vi "ReadFromDB_labelconfig.vi"(0 "DB1":T1, 5 "操作模式":T2(ring)=enum."查询数据", 7 "查询项目":string="LuxsharePN,CustomerPN,Customer,SampleDes,AWG,Length,EEPROMWrite,LabelPrint,Remarks", 11 "标识列":string, 12 "限定条件":string="where LuxsharePN='L12345678'", 13 "Page":string, 15 "Desc":string) -> (14 "数据输出2":dbl[][](array[numeric]), 16 "错误类型":string, 17 "StringArray2":string[][](array[string])=[["L12345678\t\tIBM\t40G Ethernet QSFP+ Passive DAC Cable\t28\t3000\t0\t0\trefer to IBM Spec"]], 18 "列内对数":i32=1, 19 "返回记录数目":i32=1, 20 "ConvertToArray":string[][](array[string])=[["L12345678", "", "IBM", "40G Ethernet QSFP+ Passive DAC Cable", "28", "3000", "0", "0", "refer to IBM Spec"]], 21 "status":bool, 23 "ResultString":string="L12345678\t\tIBM\t40G Ethernet QSFP+ Passive DAC Cable\t28\t3000\t0\t0\trefer to IBM Spec\r", 24 "ConvertToClusterArray":cluster{"项":string, "值":string}[](array[cluster])=[{"项"="", "值"=""}, {"项"="L12345678", "值"="L12345678"}], 25 "DataPair":dbl[](array[numeric]), 27 "数据输出":dbl[][](array[numeric]))   [LabVIEW 2011]
uses:
  <vilib>/Utility/file.llb/Read From Spreadsheet File (string).vi
  <vilib>/Utility/file.llb/Write To Spreadsheet File (string).vi
panel:
  out "result string":string="select LuxsharePN,CustomerPN,Customer,SampleDes,AWG,Length,EEPROMWrite,LabelPrint,Remarks from project where LuxsharePN='L12345678'"
  out "替换数量":i32=9
  in  "二级分隔符":string
  in  "一级分隔符":string
  in  "表名":string="vproject"
  out "Result":bool=TRUE
  in  "InitArray1":string[][](array[string])
  in  "MoveToTail":i32=1
  in  "InitArray2":string[](array[string])
  out "错误输出":errorcluster
  in  "初始化簇数组":cluster{"项":string, "值":string}[](array[cluster])
  in  "簇元素":cluster{"项":string, "值":string}
  in  "input-db":string="HTPSDB"
  in  "input-psw":string="htps'songyy"
  in  "input-user":string="htpsuser"
  in  "input-IP":string="dg-sql-01.luxshare.com.cn"
  in  "ADODB._Recordset":refnum<k7>
  in  "ADODB._Connection":refnum<k7>
  # "列名 & 表名 查询结果"
  # "输       出"
  # "输       入"
  # "基本信息\n（）"
  # "状态灯，False表示操作成功，True表示操作失败"
  # "簇数组"
  # "限定条件，设定某个条件，输出满足该条件的数据"
  # "对数"
  # "错误类型"
  # "查询记录时才需要填写，page用于设置查询一次请求的记录数，Desc用于截断Desc条记录之前的记录"
  # "改变操作时需要修改的信息"
  # "操作模式：查询表名\n                  查询列名\n                  查询记录\n                  查询总记录\n                  查询数据"
  # "字符串"
  # "数组"
  # "查询表名时不需要输入\n\n查询列名和查询数据时要指定哪一张表"
  # "字符串数组"
  # "在查询表名和列名时不需要输入信息\n\n在查询数据时，如果要输入所有列，填入“*”，如果要查询指定的某一个列，输入该列的名称"
  # "ProjectName"
  # "EEPROMContent"
  # "LimitSpec"
  # "LabelContent"
  # "SwitchMatrix"
  # "error:\n-2147217843 登陆失败： 。\n-2147467259 要访问的数据库不存在\n-2146825267 没有数据    。\n-2146824584 对象关闭时，不允许操作\n-2147217865 表名不存在 。\n-2147467259 服务器连接失败 。"
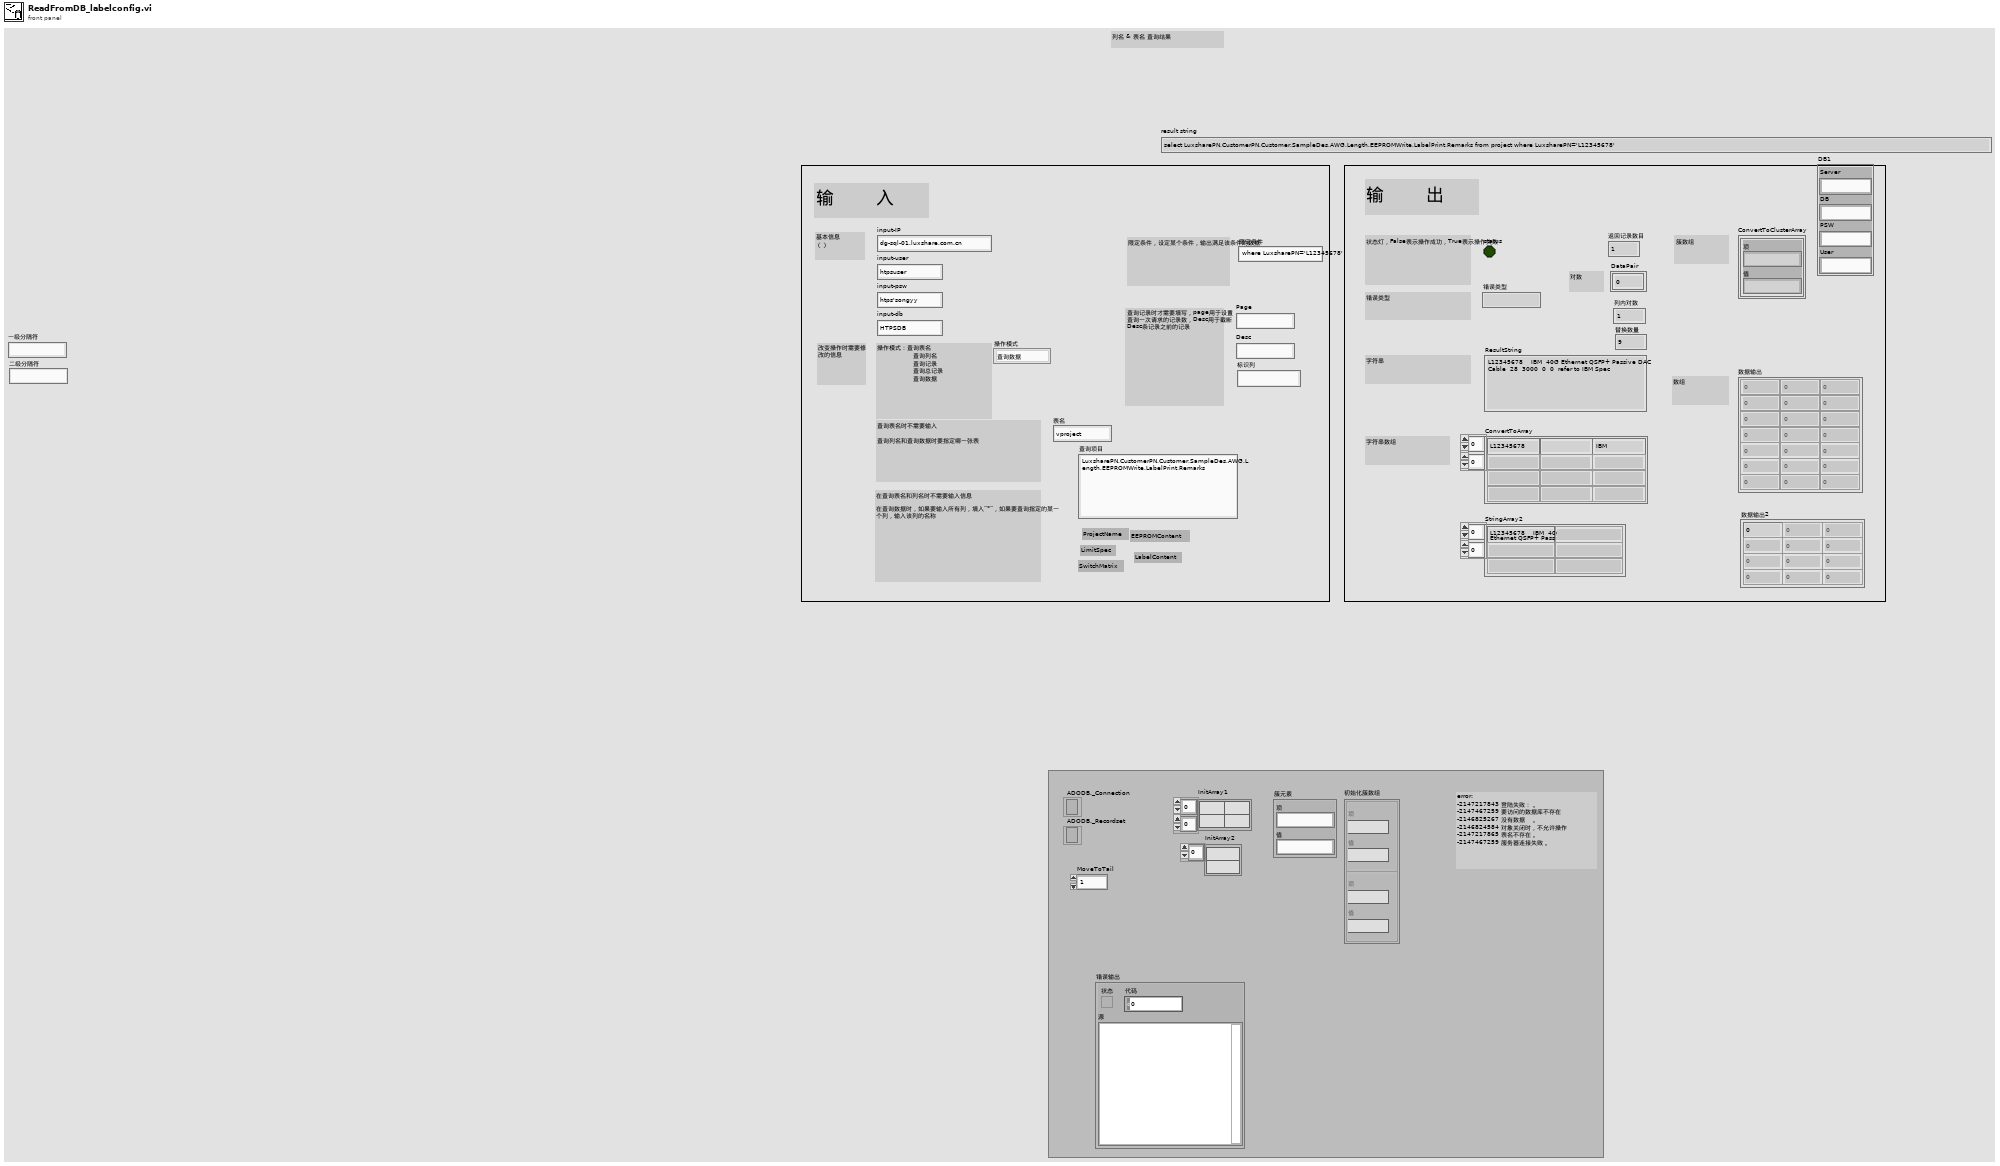
[diagram p1: front panel]
types:
  T1 = cluster{"Server":string, "DB":string, "PSW":string, "User":string}
  T2 = enum16{"查询表名", "查询列名", "查询记录", "查询总记录", "查询数据", "转换数据"}
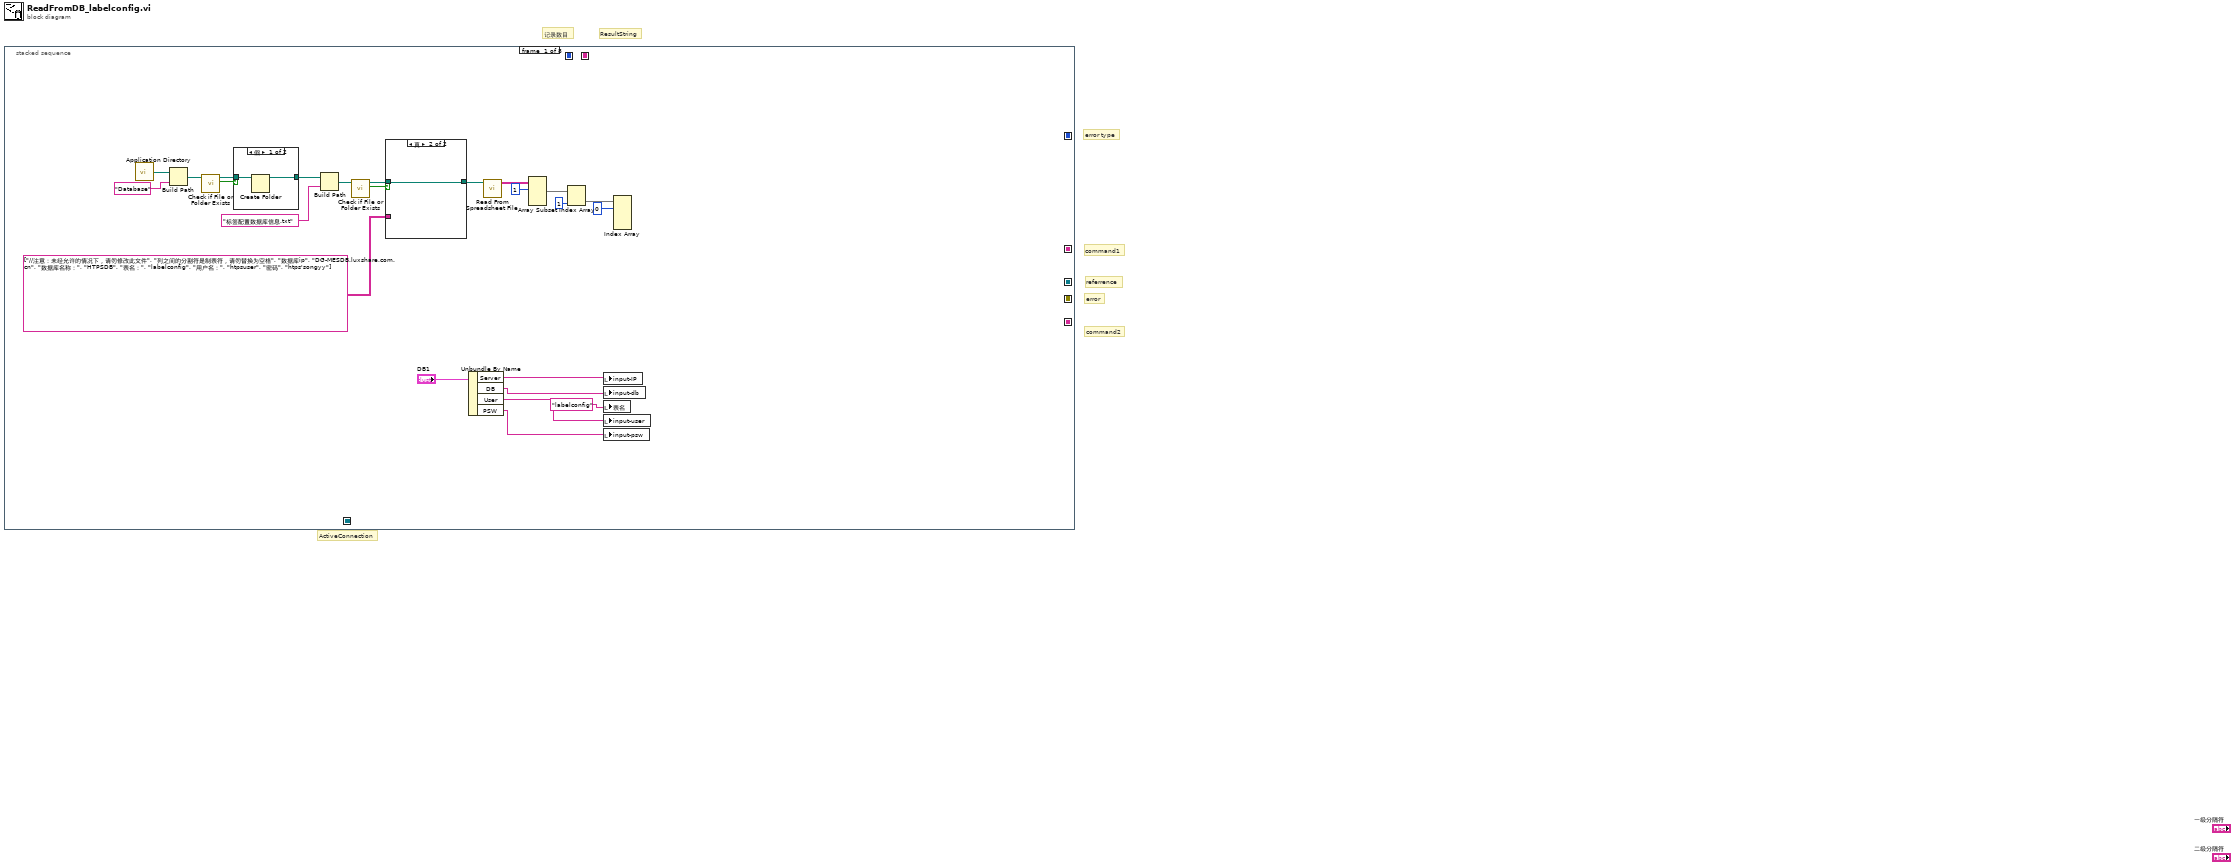
[diagram p0: block diagram]
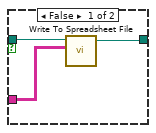
[diagram p2: hidden frame]
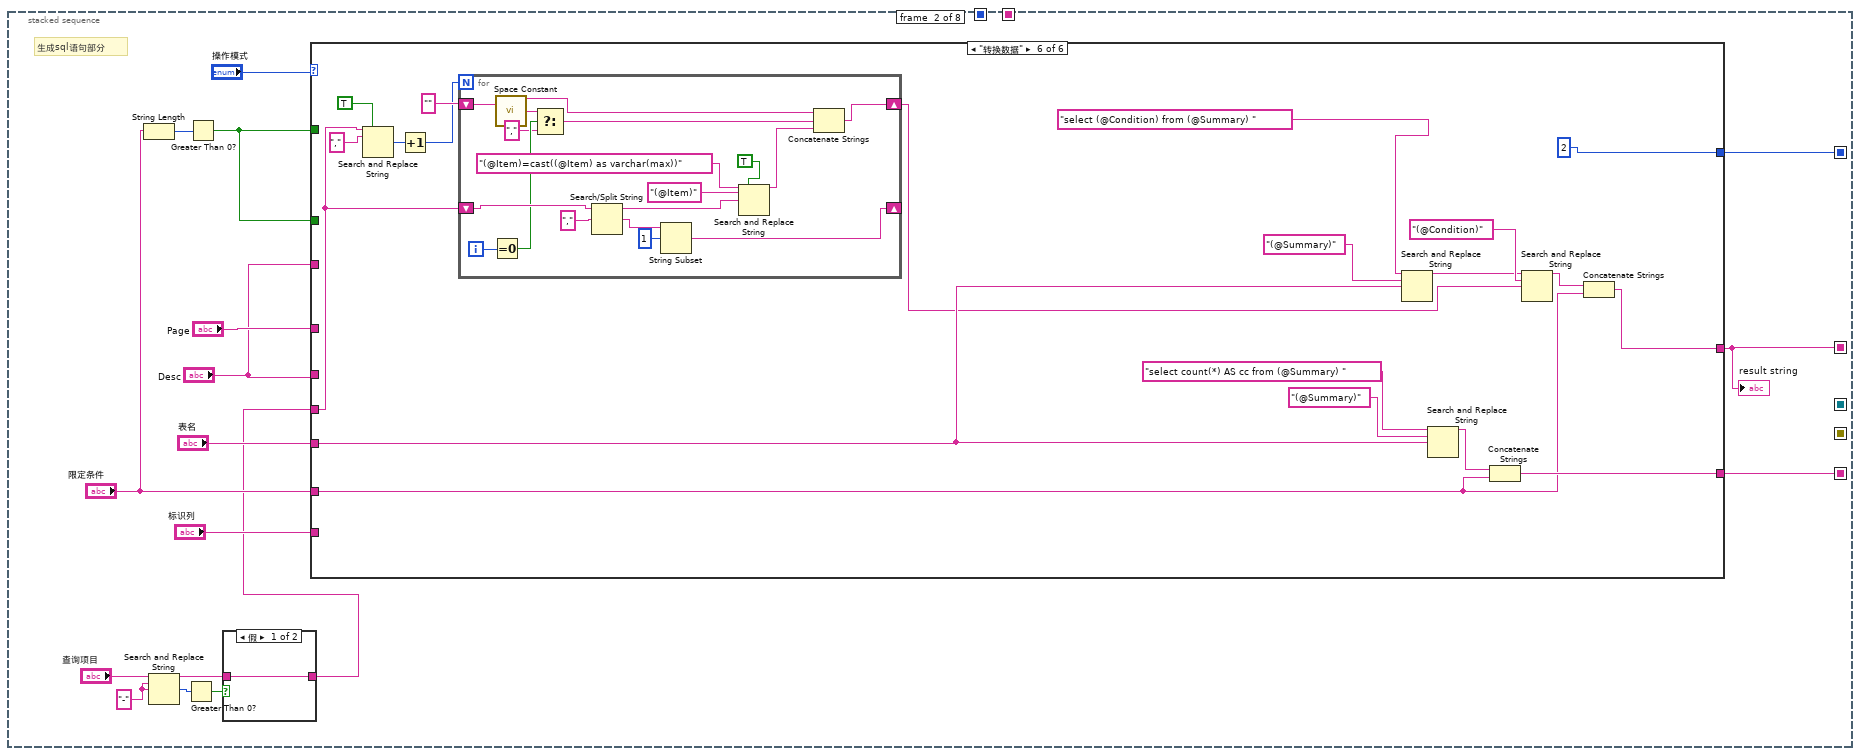
[diagram p4: hidden frame]
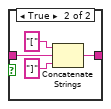
[diagram p5: hidden frame]
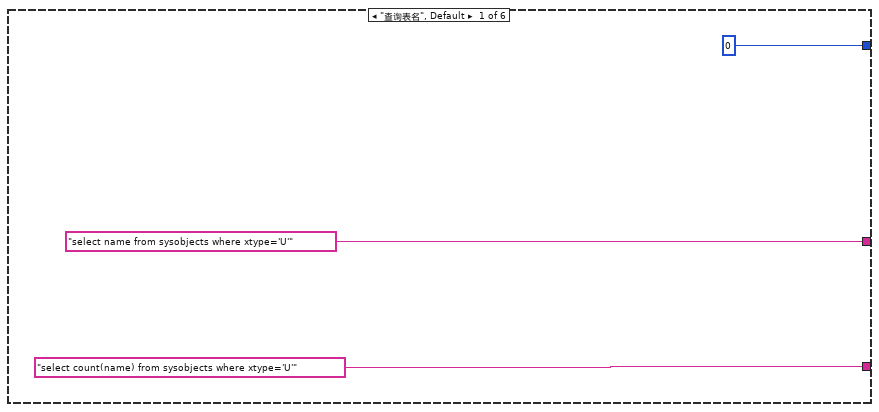
[diagram p6: hidden frame]
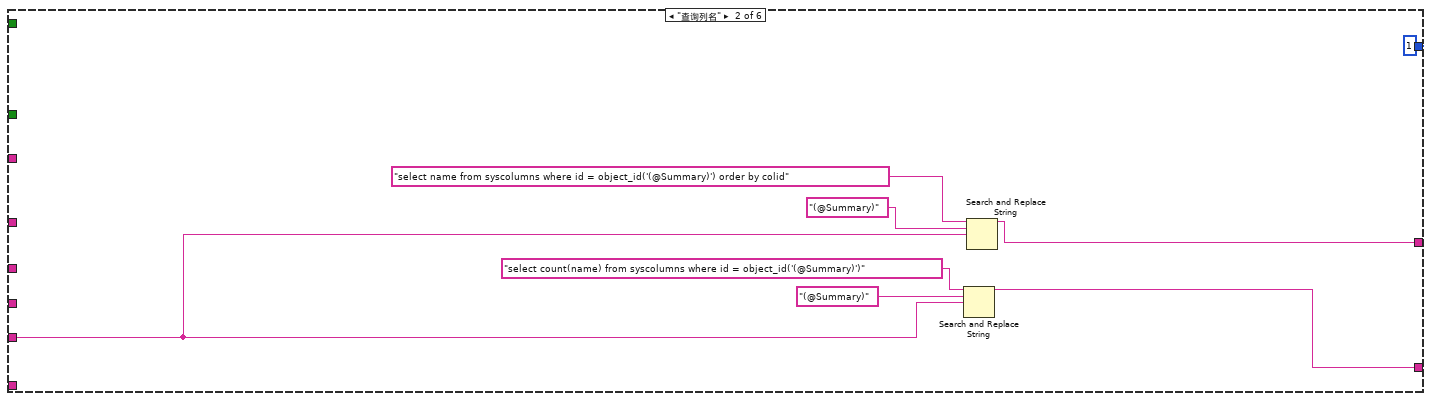
[diagram p7: hidden frame]
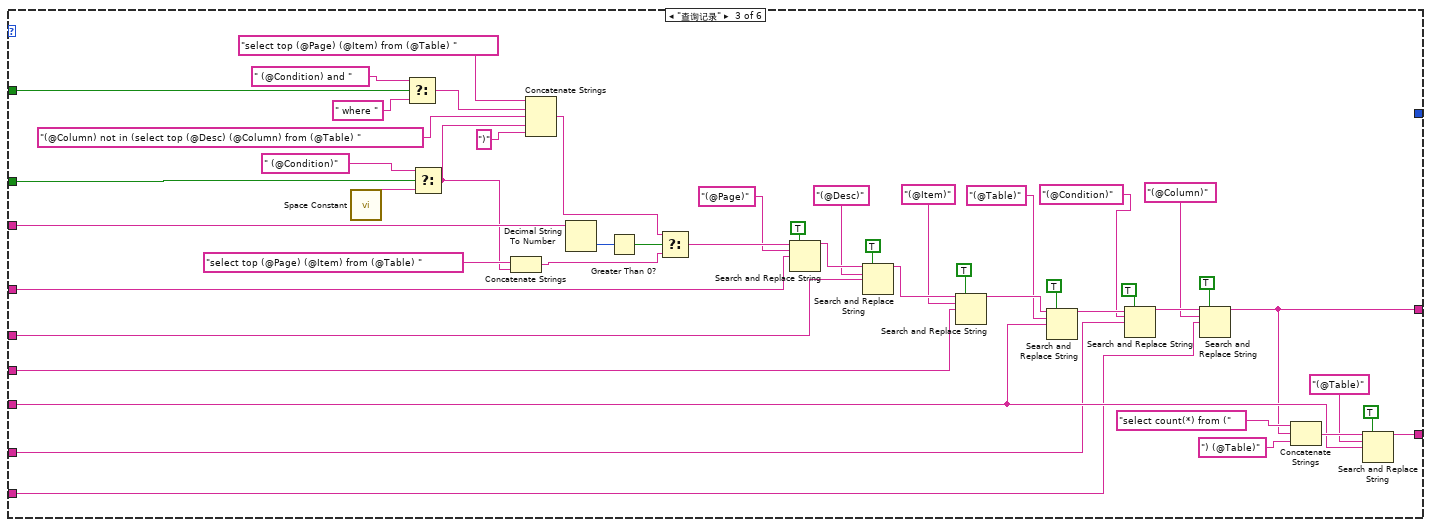
[diagram p8: hidden frame]
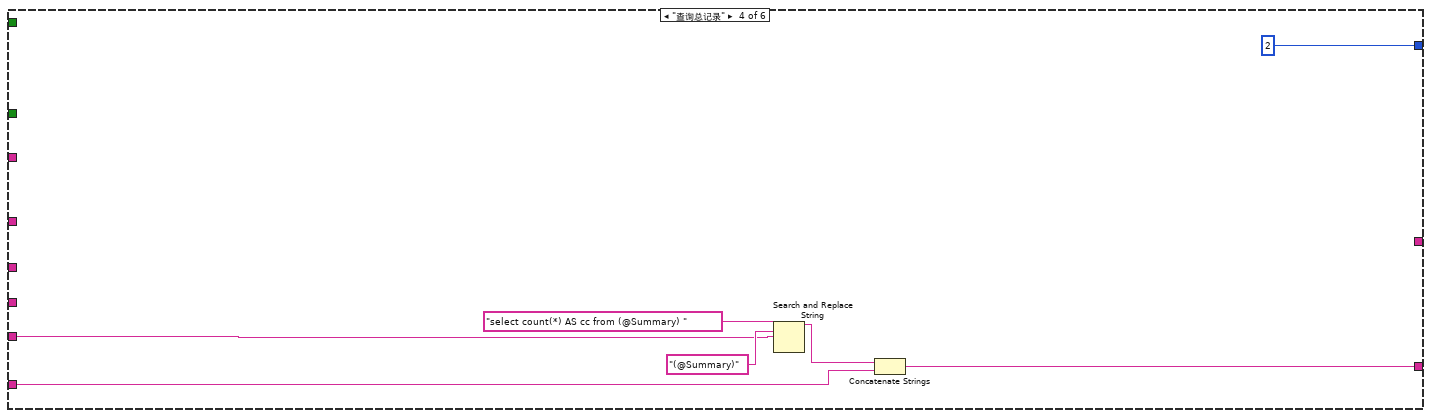
[diagram p9: hidden frame]
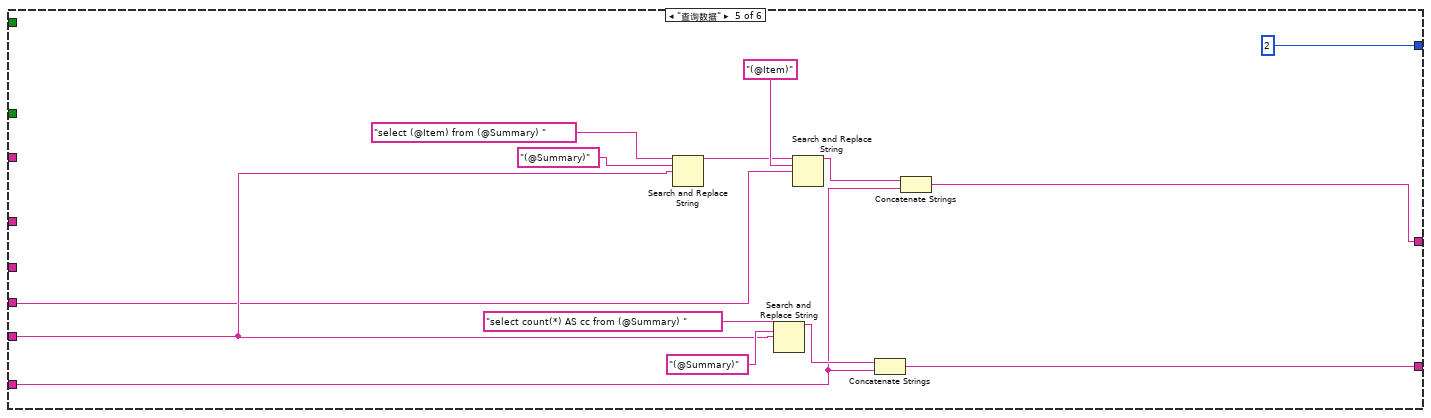
[diagram p10: hidden frame]
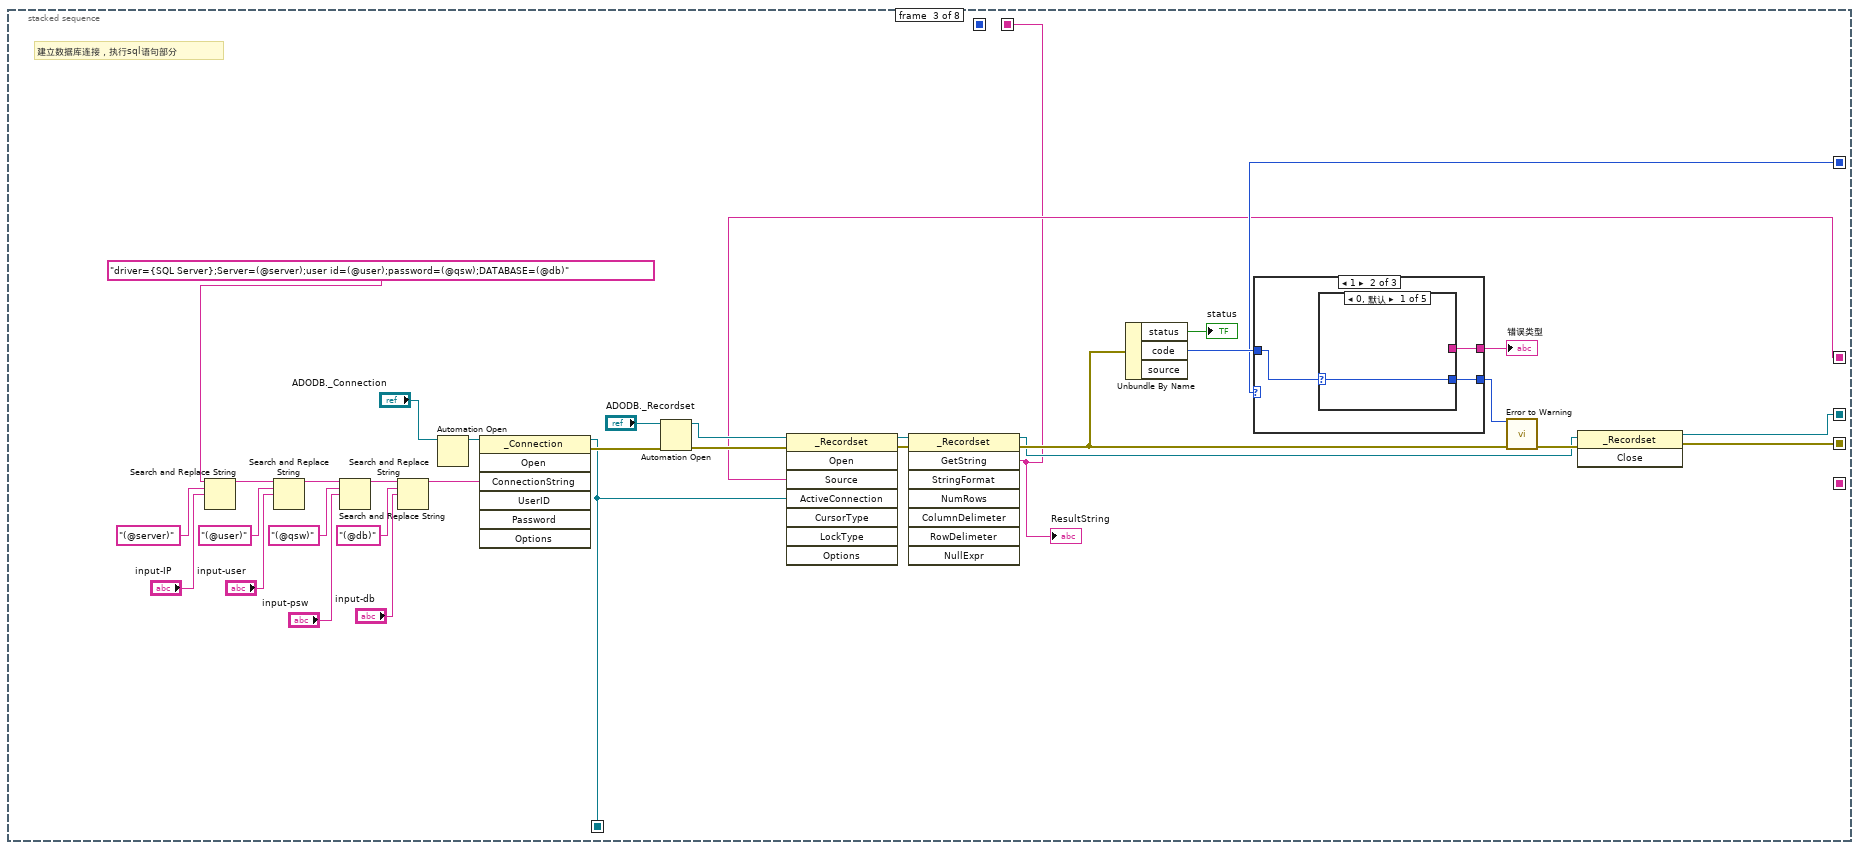
[diagram p11: hidden frame]
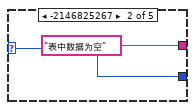
[diagram p13: hidden frame]
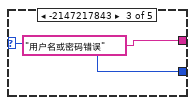
[diagram p14: hidden frame]
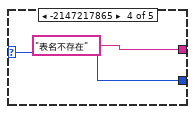
[diagram p15: hidden frame]
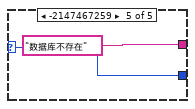
[diagram p16: hidden frame]
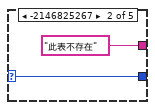
[diagram p17: hidden frame]
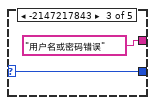
[diagram p18: hidden frame]
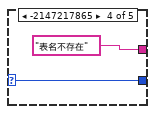
[diagram p19: hidden frame]
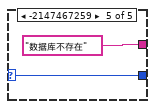
[diagram p20: hidden frame]
diagram:
  # "记录数目"
  # "ActiveConnection"
  # "referrence"
  # "error"
  # "error type"
  # "command2"
  # "command1"
  # "ResultString"
  n1 = stacked-sequence {
    seq-local: [_ _ w174 _ _ _ _ _] -> [_ _ _ w244 _ _ _ w429]
    seq-local: [_ w36 _ _ _ _ _ _] -> [_ _ w176 _ _ _ _ _]
    seq-local: [_ w35 _ _ _ _ _ _] -> [_ _ w175 _ _ _ _ _]
    seq-local: [_ _ w173 _ _ _ _ _] -> [_ _ _ _ w265 w329 w385 _]
    seq-local: [_ _ w172 _ _ _ _ _] -> [_ _ _ w242 _ _ _ _]
    seq-local: [_ _ w171 _ _ _ _ _] -> [_ _ _ w243 _ _ _ _]
    seq-local: [_ w34 _ _ _ _ _ _] -> [_ _ _ w245 _ _ _ _]
    seq-local: [_ _ _ w241 _ _ _ _] -> [_ _ _ _ w266 _ _ _]
    frame #0 {
      n2 = call <vilib>:"Application Directory.vi"() -> ("Application Directory"=w24:path)
      n3 = Build Path(base path=w24, name or relative path="Database" ("名称或相对路径")) -> (appended path=w22:path)
      n4 = call <vilib>:"Check if File or Folder Exists.vi"("path"=w22) -> ("file or folder exists?"=w21:bool, "dup path"=w20:path)  [unwired: 8 in, 1 out]
      n5 = case shown="假" w21 {
        tunnel: w20 -> [w30 w31]
        tunnel: [w29 w31] -> w19
        frame False {
          n6 = Create Folder(path (use dialog)=w30) -> (created path=w29:path)  [unwired: 2 in, 2 out]
        }
        frame True {
        }
      }
      n7 = Build Path(base path=w19, name or relative path="标签配置数据库信息.txt" ("名称或相对路径")) -> (appended path=w17:path)
      n8 = call <vilib>:"Check if File or Folder Exists.vi"("path"=w17) -> ("file or folder exists?"=w15:bool, "dup path"=w16:path)  [unwired: 8 in, 1 out]
      n9 = case shown="真" w15 {
        tunnel: w16 -> [w27 w28]
        tunnel: [w25 w28] -> w13
        tunnel: string[][] [["//注意：未经允许的情况下，请勿修改此文件", "列之间的分割符是制表符，请勿替换为空格"], ["数据库ip", "DG-MESDB.luxshare.com.cn"], ["数据库名称：", "HTPSDB"], ["表名：", "labelconfig"], ["用户名：", "htpsuser"], ["密码", "htps'songyy"]] -> [w26 _]
        frame False {
          n10 = call-poly <vilib>:"Write To Spreadsheet File.vi"("2D data"=w26, "file path (dialog if empty)"=w27) -> ("new file path (Not A Path if cancelled)"=w25:path)  [unwired: 6 in]
        }
        frame True {
        }
      }
      n11 = Unbundle By Name("DB1") -> ("Server"=w5:string, "DB"=w4:string, "User"=w2:string, "PSW"=w3:string)
      n12 = call-poly <vilib>:"Read From Spreadsheet File.vi"("file path (dialog if empty)"=w13) -> ("all rows"=w12:string[][])  [unwired: 6 in, 4 out]
      n13 = Array Subset(array=w12, index (row)=1 ("索引")) -> (w10:string[][])  [unwired: 3 in]
      n14 = Index Array(array=w10, index (col)=1 ("禁用的索引 (列)")) -> (element=w8:string[])  [unwired: 1 in]
      n15 = local write "input-IP"(w5) -> ()
      n16 = local write "input-db"(w4) -> ()
      n17 = local write "表名"("labelconfig") -> ()
      n18 = local write "input-user"(w2) -> ()
      n19 = local write "input-psw"(w3) -> ()
      n20 = Index Array(array=w8, index #1=0 ("索引")) -> ()  [unwired: 4 in, 5 out]
    }
    frame #1 {
      w46 = "-"
      # "生成sql语句部分"
      n21 = String Length(string="限定条件") -> (length=w38:i32)
      n22 = Search and Replace String(input string="查询项目", search string=w46, replace string=w46) -> (result string=w43:string, number of replacements=w45:i32)  [unwired: 5 in, 2 out]
      n23 = Greater Than 0?(x=w45) -> (x > 0?=w44:bool)
      n24 = Greater Than 0?(x=w38) -> (x > 0?=w37:bool)
      n25 = case shown="假" w44 {
        tunnel: w43 -> [w49 w52]
        tunnel: [w49 w50] -> w32
        frame False {
        }
        frame True {
          n26 = Concatenate Strings("[", w52, "]") -> (w50:string)
        }
      }
      n27 = case shown="\"转换数据\"" "操作模式" {
        tunnel: "表名" -> [_ w61 w98 w117 w130 w142]
        tunnel: "限定条件" -> [_ _ w91 w114 w122 w145]
        tunnel: ["select name from sysobjects where xtype='U'" w59 w69 _ w123 w146] -> w35
        tunnel: ["select count(name) from sysobjects where xtype='U'" w60 w97 w115 w128 w150] -> w34
        tunnel: w32 -> [_ _ w103 _ w126 w135]
        tunnel: [0 1 _ 2 2 2] -> w36
        tunnel: "Page" -> [_ _ w110 _ _ _]
        tunnel: "Desc" -> [_ _ w109 _ _ _]
        tunnel: "Desc" -> [_ _ w89 _ _ _]
        tunnel: w37 -> [_ _ w85 _ _ _]
        tunnel: w37 -> [_ _ w81 _ _ _]
        tunnel: "标识列" -> [_ _ w65 _ _ _]
        frame "查询表名", Default {
        }
        frame "查询列名" {
          n28 = Search and Replace String(input string="select count(name) from syscolumns where id = object_id('(@Summary)')", search string="(@Summary)" ("搜索字符串"), replace string=w61) -> (result string=w60:string)  [unwired: 5 in, 3 out]
          n29 = Search and Replace String(input string="select name from syscolumns where id = object_id('(@Summary)') order by colid", search string="(@Summary)" ("搜索字符串"), replace string=w61) -> (result string=w59:string)  [unwired: 5 in, 3 out]
        }
        frame "查询记录" {
          n30 = call <vilib>:"Space Constant.vi"() -> ("String"=w82:string)
          n31 = Select(t=" (@Condition) and ", s=w85, f=" where ") -> (s? t:f=w79:string)
          n32 = Select(t=" (@Condition)", s=w81, f=w82) -> (s? t:f=w74:string)
          n33 = Concatenate Strings("select top (@Page) (@Item) from (@Table) ", w74) -> (w73:string)
          n34 = Concatenate Strings("select top (@Page) (@Item) from (@Table) ", w79, "(@Column) not in (select top (@Desc) (@Column) from (@Table) ", w74, ")") -> (w76:string)
          n35 = Decimal String To Number(string=w89) -> (number=w88:i32)  [unwired: 2 in, 1 out]
          n36 = Greater Than 0?(x=w88) -> (x > 0?=w87:bool)
          n37 = Select(t=w76, s=w87, f=w73) -> (s? t:f=w86:string)
          n38 = Search and Replace String(replace all?=TRUE ("替换全部？(F)"), input string=w86, search string="(@Page)" ("搜索字符串"), replace string=w110) -> (result string=w112:string)  [unwired: 4 in, 3 out]
          n39 = Search and Replace String(replace all?=TRUE ("替换全部？(F)"), input string=w112, search string="(@Desc)" ("搜索字符串"), replace string=w109) -> (result string=w106:string)  [unwired: 4 in, 3 out]
          n40 = Search and Replace String(replace all?=TRUE ("替换全部？(F)"), input string=w106, search string="(@Item)" ("搜索字符串"), replace string=w103) -> (result string=w101:string)  [unwired: 4 in, 3 out]
          n41 = Search and Replace String(replace all?=TRUE ("替换全部？(F)"), input string=w101, search string="(@Table)" ("搜索字符串"), replace string=w98) -> (result string=w93:string)  [unwired: 4 in, 3 out]
          n42 = Search and Replace String(replace all?=TRUE ("替换全部？(F)"), input string=w93, search string="(@Condition)" ("搜索字符串"), replace string=w91) -> (result string=w68:string)  [unwired: 4 in, 3 out]
          n43 = Search and Replace String(replace all?=TRUE ("替换全部？(F)"), input string=w68, search string="(@Column)" ("搜索字符串"), replace string=w65) -> (result string=w69:string)  [unwired: 4 in, 3 out]
          n44 = Concatenate Strings("select count(*) from (", w69, ") (@Table)") -> (w100:string)
          n45 = Search and Replace String(replace all?=TRUE ("替换全部？(F)"), input string=w100, search string="(@Table)" ("搜索字符串"), replace string=w98) -> (result string=w97:string)  [unwired: 4 in, 3 out]
        }
        frame "查询总记录" {
          n46 = Search and Replace String(input string="select count(*) AS cc from (@Summary) ", search string="(@Summary)" ("搜索字符串"), replace string=w117) -> (result string=w116:string)  [unwired: 5 in, 3 out]
          n47 = Concatenate Strings(w116, w114) -> (w115:string)
        }
        frame "查询数据" {
          n48 = Search and Replace String(input string="select (@Item) from (@Summary) ", search string="(@Summary)" ("搜索字符串"), replace string=w130) -> (result string=w124:string)  [unwired: 5 in, 3 out]
          n49 = Search and Replace String(input string="select count(*) AS cc from (@Summary) ", search string="(@Summary)" ("搜索字符串"), replace string=w130) -> (result string=w129:string)  [unwired: 5 in, 3 out]
          n50 = Search and Replace String(input string=w124, search string="(@Item)" ("搜索字符串"), replace string=w126) -> (result string=w125:string)  [unwired: 5 in, 3 out]
          n51 = Concatenate Strings(w129, w122) -> (w128:string)
          n52 = Concatenate Strings(w125, w122) -> (w123:string)
        }
        frame "转换数据" {
          n53 = Search and Replace String(replace all?=TRUE ("替换全部？(F)"), input string=w135, search string="," ("搜索字符串")) -> (number of replacements=w138:i32)  [unwired: 5 in, 3 out]
          n54 = Increment(x=w138) -> (x+1=w139:i32)
          n55 = for {
            N: w139 -> [_]
            shift-right: [w157] -> w136
            shift-left: "" -> [w158]
            shift-right: [w154] -> _
            shift-left: w135 -> [w169]
            i -> [w164]
            n56 = Equal To 0?(x=w164) -> (x = 0?=w163:bool)
            n57 = call <vilib>:"Space Constant.vi"() -> ("String"=w162:string)
            n58 = Select(t=w162, s=w163, f=",") -> (s? t:f=w160:string)
            n59 = Search/Split String(string=w169, search string/char (-)="," ("搜索字符串/字符(-)")) -> (substring before match=w166:string, match + rest of string=w156:string)  [unwired: 1 in, 1 out]
            n60 = String Subset(string=w156, offset (0)=1 ("偏移量(0)")) -> (substring=w154:string)  [unwired: 1 in]
            n61 = Search and Replace String(replace all?=TRUE ("替换全部？(F)"), input string="(@Item)=cast((@Item) as varchar(max))", search string="(@Item)", replace string=w166) -> (result string=w159:string)  [unwired: 4 in, 3 out]
            n62 = Concatenate Strings(w158, w160, w159) -> (w157:string)
          }
          n63 = Search and Replace String(input string="select (@Condition) from (@Summary) ", search string="(@Summary)" ("搜索字符串"), replace string=w142) -> (result string=w147:string)  [unwired: 5 in, 3 out]
          n64 = Search and Replace String(input string="select count(*) AS cc from (@Summary) ", search string="(@Summary)" ("搜索字符串"), replace string=w142) -> (result string=w151:string)  [unwired: 5 in, 3 out]
          n65 = Concatenate Strings(w151, w145) -> (w150:string)
          n66 = Search and Replace String(input string=w147, search string="(@Condition)" ("搜索字符串"), replace string=w136) -> (result string=w148:string)  [unwired: 5 in, 3 out]
          n67 = Concatenate Strings(w148, w145) -> (w146:string)
        }
      }
      "result string" <- w35
    }
    frame #2 {
      # "建立数据库连接，执行sql语句部分"
      n68 = Search and Replace String(input string="driver={SQL Server};Server=(@server);user id=(@user);password=(@qsw);DATABASE=(@db)" ("ConnectionString"), search string="(@server)" ("搜索字符串"), replace string="input-IP") -> (result string=w181:string)  [unwired: 5 in, 3 out]
      n69 = Search and Replace String(input string=w181, search string="(@user)" ("搜索字符串"), replace string="input-user") -> (result string=w184:string)  [unwired: 5 in, 3 out]
      n70 = Search and Replace String(input string=w184, search string="(@qsw)" ("搜索字符串"), replace string="input-psw") -> (result string=w187:string)  [unwired: 5 in, 3 out]
      n71 = Search and Replace String(input string=w187, search string="(@db)" ("搜索字符串"), replace string="input-db") -> (result string=w191:string)  [unwired: 5 in, 3 out]
      n72 = Automation Open(Automation Refnum="ADODB._Connection") -> (Automation Refnum=w177:refnum<k7>)  [unwired: 3 in, 1 out]
      n73 = invoke class="_Connection" method="Open"(reference=w177, "ConnectionString"=w191) -> (reference out=w174:refnum<k7>, error out=w194:errorcluster)  [unwired: 5 in, 5 out]
      n74 = Automation Open(error in (no error)=w194, Automation Refnum="ADODB._Recordset") -> (Automation Refnum=w193:refnum<k7>, error out=w195:errorcluster)  [unwired: 2 in]
      n75 = invoke class="_Recordset" method="Open"(reference=w193, error in=w195, "Source"=w175, "ActiveConnection"=w174) -> (reference out=w196:refnum<k7>, error out=w197:errorcluster)  [unwired: 4 in, 6 out]
      n76 = invoke class="_Recordset" method="GetString"(reference=w196, error in=w197) -> (reference out=w198:refnum<k7>, error out=w204:errorcluster, "GetString"=w173:string)  [unwired: 6 in, 5 out]
      "ResultString" <- w173
      n77 = Unbundle By Name(w204) -> ("status"=→"status":bool, "code"=w201:i32)  [unwired: 1 out]
      n78 = case shown="1" w176 {
        tunnel: w201 -> [w207 w219 w229]
        tunnel: [w206 w218 w231] -> w202
        tunnel: [w205 w217 w230] -> w203
        frame 0, Default {
          n79 = case shown="0, 默认" w207 {
            selector: w207 -> [w208 w210 w211 w214 w215]
            tunnel: [w208 w210 w211 w214 w215] -> w206
            tunnel: [_ "表中数据为空" "用户名或密码错误" "表名不存在" "数据库不存在"] -> w205
            frame 0, Default {
            }
            frame -2146825267 {
            }
            frame -2147217843 {
            }
            frame -2147217865 {
            }
            frame -2147467259 {
            }
          }
        }
        frame 1 {
          n80 = case shown="0, 默认" w219 {
            selector: w219 -> [w220 w222 w223 w226 w227]
            tunnel: [w220 w222 w223 w226 w227] -> w218
            tunnel: [_ "此表不存在" "用户名或密码错误" "表名不存在" "数据库不存在"] -> w217
            frame 0, Default {
            }
            frame -2146825267 {
            }
            frame -2147217843 {
            }
            frame -2147217865 {
            }
            frame -2147467259 {
            }
          }
        }
        frame 2 {
          n81 = case shown="-2147467259" w229 {
            selector: w229 -> [w232 w234 w235 w238 w239]
            tunnel: [w232 w234 w235 w238 w239] -> w231
            tunnel: [_ "表中数据为空" "用户名或密码错误" "表名不存在" "数据库不存在"] -> w230
            frame 0, Default {
            }
            frame -2146825267 {
            }
            frame -2147217843 {
            }
            frame -2147217865 {
            }
            frame -2147467259 {
            }
          }
        }
      }
      "错误类型" <- w203
      n82 = call <vilib>:"Error to Warning.vi"("1st Error to Convert"=w202, "error in"=w204) -> ("warning out"=w199:errorcluster)  [unwired: 13 in]
      n83 = invoke class="_Recordset" method="Close"(reference=w198, error in=w199) -> (reference out=w171:refnum<k7>, error out=w172:errorcluster)  [unwired: 1 in, 1 out]
    }
    frame #3 {
      # "执行sql语句部分\n此部分执行的sql语句的作用是统计返回的记录数目"
      n84 = call <vilib>:"Error to Warning.vi"("1st Error to Convert"=-2146824584, "error in"=w242) -> ("warning out"=w255:errorcluster)  [unwired: 13 in]
      n85 = invoke class="_Recordset" method="Open"(reference=w243, error in=w255, "Source"=w245, "ActiveConnection"=w244) -> (reference out=w250:refnum<k7>, error out=w254:errorcluster)  [unwired: 4 in, 6 out]
      n86 = invoke class="_Recordset" method="GetString"(reference=w250, error in=w254) -> (reference out=w252:refnum<k7>, error out=w257:errorcluster, "GetString"=w251:string)  [unwired: 6 in, 5 out]
      n87 = Decimal String To Number(string=w251) -> (number=w241:i32)  [unwired: 2 in, 1 out]
      "返回记录数目" <- w241
      n88 = call <vilib>:"Error to Warning.vi"("1st Error to Convert"=-2147217865, "error in"=w257) -> ("warning out"=w258:errorcluster)  [unwired: 13 in]
      n89 = Greater Than 0?(x=w241) -> (x > 0?=w246:bool)
      n90 = invoke class="_Recordset" method="Close"(reference=w252, error in=w258) -> (reference out=w253:refnum<k7>, error out=w261:errorcluster)  [unwired: 1 in, 1 out]
      n91 = Select(t=TRUE, s=w246, f=FALSE) -> (s? t:f=→"Result":bool)
      n92 = call <vilib>:"Error to Warning.vi"("1st Error to Convert"=-2147217864, "2nd Error to Convert"=-2147467259, "error in"=w261) -> ("warning out"=w262:errorcluster)  [unwired: 12 in]
      n93 = Close Reference(reference=w253, error in (no error)=w262) -> (error out=→"错误输出":errorcluster)
    }
    frame #4 {
      w281 = "\t"
      # "此部分对数据的处理主要针对记录"
      n94 = Search/Split String(string=w265, search string/char (-)="\r") -> (substring before match=w280:string)  [unwired: 1 in, 2 out]
      n95 = Search and Replace String(replace all?=TRUE ("替换全部？(F)"), input string=w280, search string=w281, replace string=w281) -> (number of replacements=w283:i32)  [unwired: 4 in, 3 out]
      n96 = Increment(x=w283) -> (x+1=w284:i32)
      "替换数量" <- w284
      n97 = for {
        N: w266 -> [_]
        shift-right: [w290] -> w277
        shift-left: "InitArray1" -> [w291]
        shift-right: [w287] -> _
        shift-left: w265 -> [w293]
        tunnel: w284 -> [w286]
        i -> [w288]
        n98 = Decrement(x=w286) -> (x-1=w285:i32)
        n99 = for {
          N: w286 -> [_]
          shift-right: [w302] -> w287
          shift-left: w293 -> [w306]
          shift-right: [w303] -> w289
          shift-left: "InitArray2" -> [w305]
          tunnel: w285 -> [w294]
          i -> [w299]
          n100 = Equal?(x=w299, y=w294) -> (x = y?=w298:bool)
          n101 = Select(t="return", s=w298, f="table") -> (s? t:f=w295:string)
          n102 = case shown="\"return\"" w295 {
            tunnel: ["," "" "\t" "\r" "\n" "\r\n"] -> w307
            frame "comma", Default {
            }
            frame "space" {
            }
            frame "table" {
              # "\\t"
            }
            frame "return" {
              # "\\r"
            }
            frame "newline" {
              # "\\n"
            }
            frame "lineover" {
              # "\\r\\n"
            }
          }
          n103 = Search/Split String(string=w306, search string/char (-)=w307) -> (substring before match=w304:string, match + rest of string=w301:string)  [unwired: 1 in, 1 out]
          n104 = Insert Into Array(array=w305, index=w299, new element=w304) -> (w303:string[])
          n105 = case shown="1, 默认" "MoveToTail" {
            tunnel: [w308 w310 w314] -> w302
            tunnel: w301 -> [w309 w311 w313]
            frame 1, Default {
              n106 = Rotate String(1:w309) -> (0:w308:string)
            }
            frame 2 {
              n107 = Rotate String(1:w311) -> (0:w312:string)
              n108 = Rotate String(1:w312) -> (0:w310:string)
            }
            frame 3 {
              n109 = Rotate String(1:w313) -> (0:w316:string)
              n110 = Rotate String(1:w316) -> (0:w315:string)
              n111 = Rotate String(1:w315) -> (0:w314:string)
            }
          }
        }
        n112 = Insert Into Array(array=w291, index (row)=w288, new element=w289) -> (w290:string[][])  [unwired: 1 in]
      }
      "ConvertToArray" <- w277
      n113 = Index Array(array=w277, index (col)=0 ("禁用的索引 (列)")) -> (element=w274:string[])  [unwired: 1 in]
      n114 = Array Size(array=w277) -> (size(s)=w270:i32[])
      n115 = Build Array (concatenate)("", w274) -> (w275:string[])
      n116 = Index Array(array=w270, index=0 ("索引")) -> (element=w272:i32)
      n117 = Increment(x=w272) -> (x+1=w278:i32)
      n118 = for {
        N: w278 -> [_]
        tunnel: w275 -> [w328] mode=indexing
        shift-right: [w325] -> w268
        shift-left: "初始化簇数组" -> [w326]
        i -> [w327]
        n119 = Bundle By Name(cluster="簇元素", "项"=w328, "值"=w328) -> (w323:cluster{"项":string, "值":string})
        n120 = Insert Into Array(array=w326, index=w327, new element=w323) -> (w325:cluster{"项":string, "值":string}[])
      }
      "ConvertToClusterArray" <- w268
    }
    frame #5 {
      w330 = ":" ("搜索字符串")
      # "此部分对数据处理针对具体的测量数据"
      n121 = Search and Replace String(replace all?=TRUE ("替换全部？(F)"), input string=w329, search string=w330, replace string=w330) -> (number of replacements=w332:i32)  [unwired: 4 in, 3 out]
      n122 = Increment(x=w332) -> (x+1=w337:i32)
      "列内对数" <- w337
      n123 = for {
        N: w337 -> [_]
        shift-right: [w346] -> _
        shift-left: w329 -> [w347]
        shift-right: [w344] -> w334
        shift-left: dbl[][] [] -> [w340]
        shift-right: [w338] -> w336
        shift-left: dbl[][] [] -> [w339]
        i -> [w343]
        n124 = while {
          shift-right: [w359] -> w341
          shift-left: dbl[] [] -> [w360]
          shift-right: [w361] -> w346
          shift-left: w347 -> [w362]
          i -> [w358]
          stop <- w356 stop-if-true
          n125 = while {
            shift-right: [w371] -> w361
            shift-left: w362 -> [w373]
            shift-right: [w369] -> w354
            shift-left: "" -> [w370]
            tunnel: [w367] -> w357
            stop <- w368 stop-if-true
            n126 = Search/Split String(string=w373, offset (0)=1 ("偏移量(0)")) -> (substring before match=w367:string, match + rest of string=w371:string)  [unwired: 1 in, 1 out]
            n127 = case shown="默认" w367 {
              selector: w367 -> [_ _ _ w382]
              tunnel: w370 -> [w374 w376 w379 w383]
              tunnel: [w374 w376 w379 w381] -> w369
              tunnel: [TRUE TRUE TRUE FALSE] -> w368
              frame ":" {
              }
              frame "," {
              }
              frame "" {
              }
              frame Default {
                n128 = Concatenate Strings(w383, w382) -> (w381:string)
              }
            }
          }
          n129 = Fract/Exp String To Number(string=w354) -> (number=w353:dbl)  [unwired: 3 in, 1 out]
          n130 = case shown="\",\"" w357 {
            tunnel: [TRUE FALSE TRUE TRUE] -> w356
            frame ":" {
            }
            frame "," {
            }
            frame "" {
            }
            frame Default {
            }
          }
          n131 = Insert Into Array(array=w360, index=w358, new element=w353) -> (w359:dbl[])
        }
        n132 = Greater Than 0?(x=w343) -> (x > 0?=w342:bool)
        n133 = case shown="真" w342 {
          tunnel: [w349 w352] -> w344
          tunnel: w340 -> [w349 w351]
          tunnel: w341 -> [w348 w350]
          frame False {
            "DataPair" <- w348
          }
          frame True {
            n134 = Insert Into Array(array=w351, new element=w350) -> (w352:dbl[][])  [unwired: 2 in]
          }
        }
        n135 = Insert Into Array(array=w339, new element=w341) -> (w338:dbl[][])  [unwired: 2 in]
      }
      "数据输出" <- w334
      "数据输出2" <- w336
    }
    frame #6 {
      (unwired) 0.0
      w386 = ":" ("搜索字符串")
      # "此部分对数据处理针对具体的测量数据"
      n136 = Search and Replace String(replace all?=TRUE ("替换全部？(F)"), input string=w385, search string=w386, replace string=w386) -> (number of replacements=w388:i32)  [unwired: 4 in, 3 out]
      n137 = Increment(x=w388) -> (x+1=w390:i32)
      n138 = for {
        N: w390 -> [_]
        shift-right: [w396] -> _
        shift-left: w385 -> [w397]
        shift-right: [w391] -> w384
        shift-left: string[][] [] -> [w392]
        i -> [w394]
        n139 = Greater Than 0?(x=w394) -> ()  [unwired: 1 out]
        n140 = while {
          shift-right: [w404] -> w393
          shift-left: string[] [] -> [w405]
          shift-right: [w406] -> w396
          shift-left: w397 -> [w407]
          i -> [w403]
          stop <- w401 stop-if-true
          n141 = while {
            shift-right: [w416] -> w406
            shift-left: w407 -> [w418]
            shift-right: [w414] -> w399
            shift-left: "" -> [w415]
            tunnel: [w412] -> w402
            stop <- w413 stop-if-true
            n142 = Search/Split String(string=w418, offset (0)=1 ("偏移量(0)")) -> (substring before match=w412:string, match + rest of string=w416:string)  [unwired: 1 in, 1 out]
            n143 = case shown="\"\"" w412 {
              selector: w412 -> [_ _ _ w427]
              tunnel: w415 -> [w419 w421 w424 w428]
              tunnel: [w419 w421 w424 w426] -> w414
              tunnel: [TRUE TRUE TRUE FALSE] -> w413
              frame ":" {
              }
              frame "," {
              }
              frame "" {
              }
              frame Default {
                n144 = Concatenate Strings(w428, w427) -> (w426:string)
              }
            }
          }
          n145 = call <vilib>:"Trim Whitespace.vi"("string"=w399) -> ("trimmed string"=w398:string)  [unwired: 1 in]
          n146 = case shown="\",\"" w402 {
            tunnel: [TRUE FALSE TRUE TRUE] -> w401
            frame ":" {
            }
            frame "," {
            }
            frame "" {
            }
            frame Default {
            }
          }
          n147 = Insert Into Array(array=w405, index=w403, new element=w398) -> (w404:string[])
        }
        n148 = Insert Into Array(array=w392, new element=w393) -> (w391:string[][])  [unwired: 2 in]
      }
      "StringArray2" <- w384
    }
    frame #7 {
      n149 = invoke class="_Connection" method="Close"(reference=w429) -> ()  [unwired: 2 in, 3 out]
    }
  }
